vi "Get IP.vi"() -> (2 "IP Address":string, 5 "IP Address(Bytes)":u8[](array[numeric]))   [LabVIEW 2014, in "SSL Lib.lvlib"]
doc: "VI Function: This VI gives the IP address of the localhost.\n\nVI Version: 1.0\n\nVI Author: Runjhun Agarwal"
uses:
  <userlib>/SSL Library/SSL Lib.lvlib
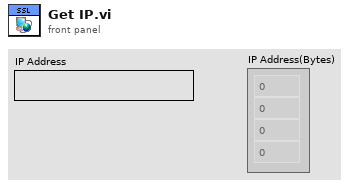
[diagram p1: front panel]
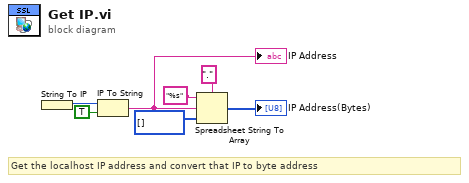
[diagram p0: block diagram]
diagram:
  # "Get the localhost IP address and convert that IP to byte address"
  n1 = String To IP() -> (0:w7:u32)  [unwired: 1 in]
  n2 = IP To String(1:TRUE ("dot notation? (F)"), 2:w7) -> (0:w3:string)
  "IP Address" <- w3
  n3 = Spreadsheet String To Array(delimiter (Tab)=".", format string="%s", spreadsheet string=w3, array type (2D Dbl)=u8[] [] ("address")) -> (array=→"IP Address(Bytes)":u8[])
